vi "Close Interface.vi"(8 "error in (no error)":errorcluster) -> (0 "error out":errorcluster)   [LabVIEW 2019, in "Camera Engine.lvlib"]
uses:
  Camera Engine.lvlib
  <userlib>/JUL/Interface Module/Interface Library/Interface.lvlib
  <userlib>/JUL/Interface Module/Interface Library/Abort VI(VI Refnum)(Single).vi
panel:
  # "Input"
  # "Output"
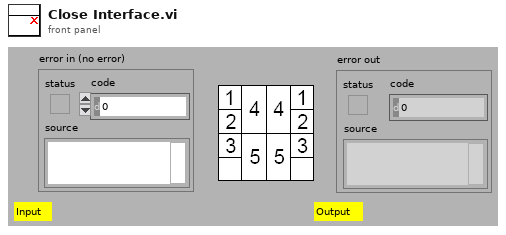
[diagram p1: front panel]
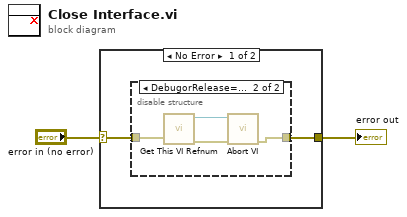
[diagram p0: block diagram]
diagram:
  n1 = case shown="No Error" "error in (no error)" {
    selector: "error in (no error)" -> [w3 w10]
    tunnel: [w4 w10] -> w1
    frame No Error {
      n2 = disable-structure shown="DebugorRelease==Release" {
        disable-tunnel: [w5 w6] -> w4
        disable-tunnel: w3 -> [w5 w9]
        frame condition #0 (active) {
        }
        frame condition #1 {
          n3 = call "Get This VI Refnum.vi"("error in (no error)"=w9) -> ("error out"=w8:errorcluster, "This VI Refnum Out"=w7:refnum<vi>)  [unwired: 9 in]
          n4 = call-poly <userlib>:"Abort VI.vi"("error in (no error)"=w8, "VI Refnum"=w7) -> ("error out"=w6:errorcluster)  [unwired: 9 in]
        }
      }
    }
    frame Error {
    }
  }
  "error out" <- w1
